vi "Instr_InitObject.vi"(8 "error in (no error)":errorcluster, 9 "Instrument Configuration":variant, 10 "GPIB Address":string, 11 "InstrControl in":refnum<class "InstrControl.lvclass">) -> (0 "error out":errorcluster, 3 "InstrControl out":refnum<class "InstrControl.lvclass">)   [LabVIEW 2019, in "InstrControl.lvclass"]
uses:
  InstrControl.lvclass
  InstrControl.lvclass/InstrControl.ctl
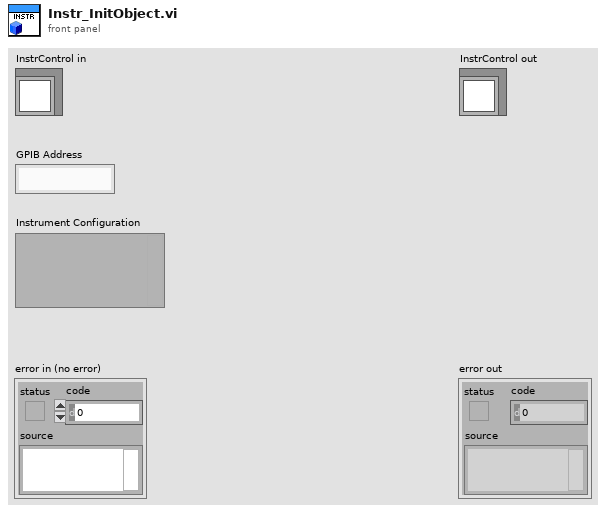
[diagram p1: front panel]
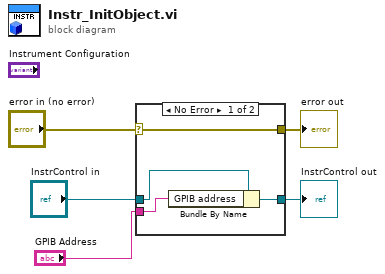
[diagram p0: block diagram]
diagram:
  n1 = case shown="No Error" "error in (no error)" {
    selector: "error in (no error)" -> [w9 w11]
    tunnel: [w9 w11] -> w4
    tunnel: [w7 w10] -> w2
    tunnel: "InstrControl in" -> [w8 w10]
    tunnel: "GPIB Address" -> [w6 _]
    frame No Error {
      n2 = Bundle By Name(cluster=w8, "GPIB address"=w6) -> (w7:refnum<class "InstrControl.lvclass">)
    }
    frame Error {
    }
  }
  "error out" <- w4
  "InstrControl out" <- w2
